vi "relative movement.vi"(3 "representative width between wheels":dbl, 4 "speeds":cluster{"right speed":dbl, "left speed":dbl} {"left speed" step=0.05000000074505806 scale=-1.0..1.0; "right speed" step=0.05000000074505806 scale=-1.0..1.0}, 5 "start direction":dbl) -> (0 "right position":cluster{dbl, dbl}, 1 "left position":cluster{dbl, dbl}, 2 "direction":dbl)   [LabVIEW 2009]
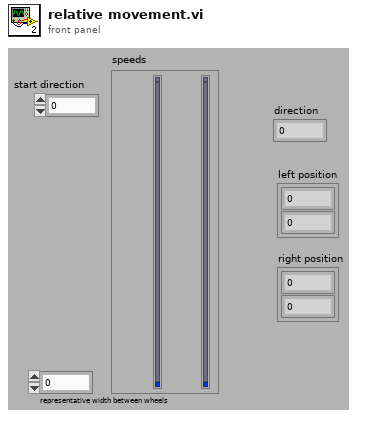
[diagram p1: front panel]
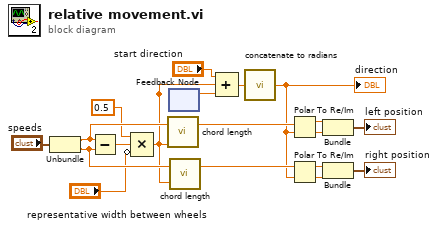
[diagram p0: block diagram]
diagram:
  n1 = Unbundle("speeds") -> ("right speed"=w8:dbl, "left speed"=w9:dbl)
  n2 = Subtract(x=w8, y=w9) -> (x-y=w2:dbl)
  n3 = Compound Arithmetic op=MULTIPLY(0.5, w2, invert "representative width between wheels") -> (w5:dbl)
  n4 = call "chord length.vi"("theta"=w5, "arc length"=w8) -> ("chord length"=w16:dbl)  [unwired: 1 in]
  n5 = feedback #1() -> (w3:dbl)  [unwired: 1 in]
  n6 = call "chord length.vi"("theta"=w5, "arc length"=w9) -> ("chord length"=w17:dbl)  [unwired: 1 in]
  n7 = Compound Arithmetic op=ADD("start direction", w5, w3) -> (w1:dbl)
  n8 = call "concatenate to radians.vi"("value"=w1) -> ("concatenated value"=w14:dbl)
  "direction" <- w14
  n9 = Polar To Re/Im(2:w14, 3:w16) -> (0:w12:dbl, 1:w11:dbl)
  n10 = Polar To Re/Im(2:w14, 3:w17) -> (0:w13:dbl, 1:w15:dbl)
  n11 = Bundle(w11, w12) -> (→"left position":cluster{dbl, dbl})  [unwired: 1 in]
  n12 = Bundle(w15, w13) -> (→"right position":cluster{dbl, dbl})  [unwired: 1 in]
